vi "DAQAssist-SimulatedSignal.vi"(0 "reference":refnum<vi>, 1 "Stbd Cluster":T2, 2 "Port Cluster":T2, 3 "Corner Cluster Stbd":T1, 4 "Corner Cluster Port":T1) -> (5 "Dynamic Data":dynamicdata(waveform))   [LabVIEW 2012]
uses:
  <vilib>/Analysis/NI_AALPro.lvlib
panel:
  out "x*y":dbl[](array[numeric])
  out "Waveform Graph 2":dynamicdata(graph)
  out "Waveform Graph 3":dynamicdata(graph)
  out "Waveform Graph":dynamicdata(graph)
  out "Frequency Port":dbl
  out "Frequency Stbd":dbl
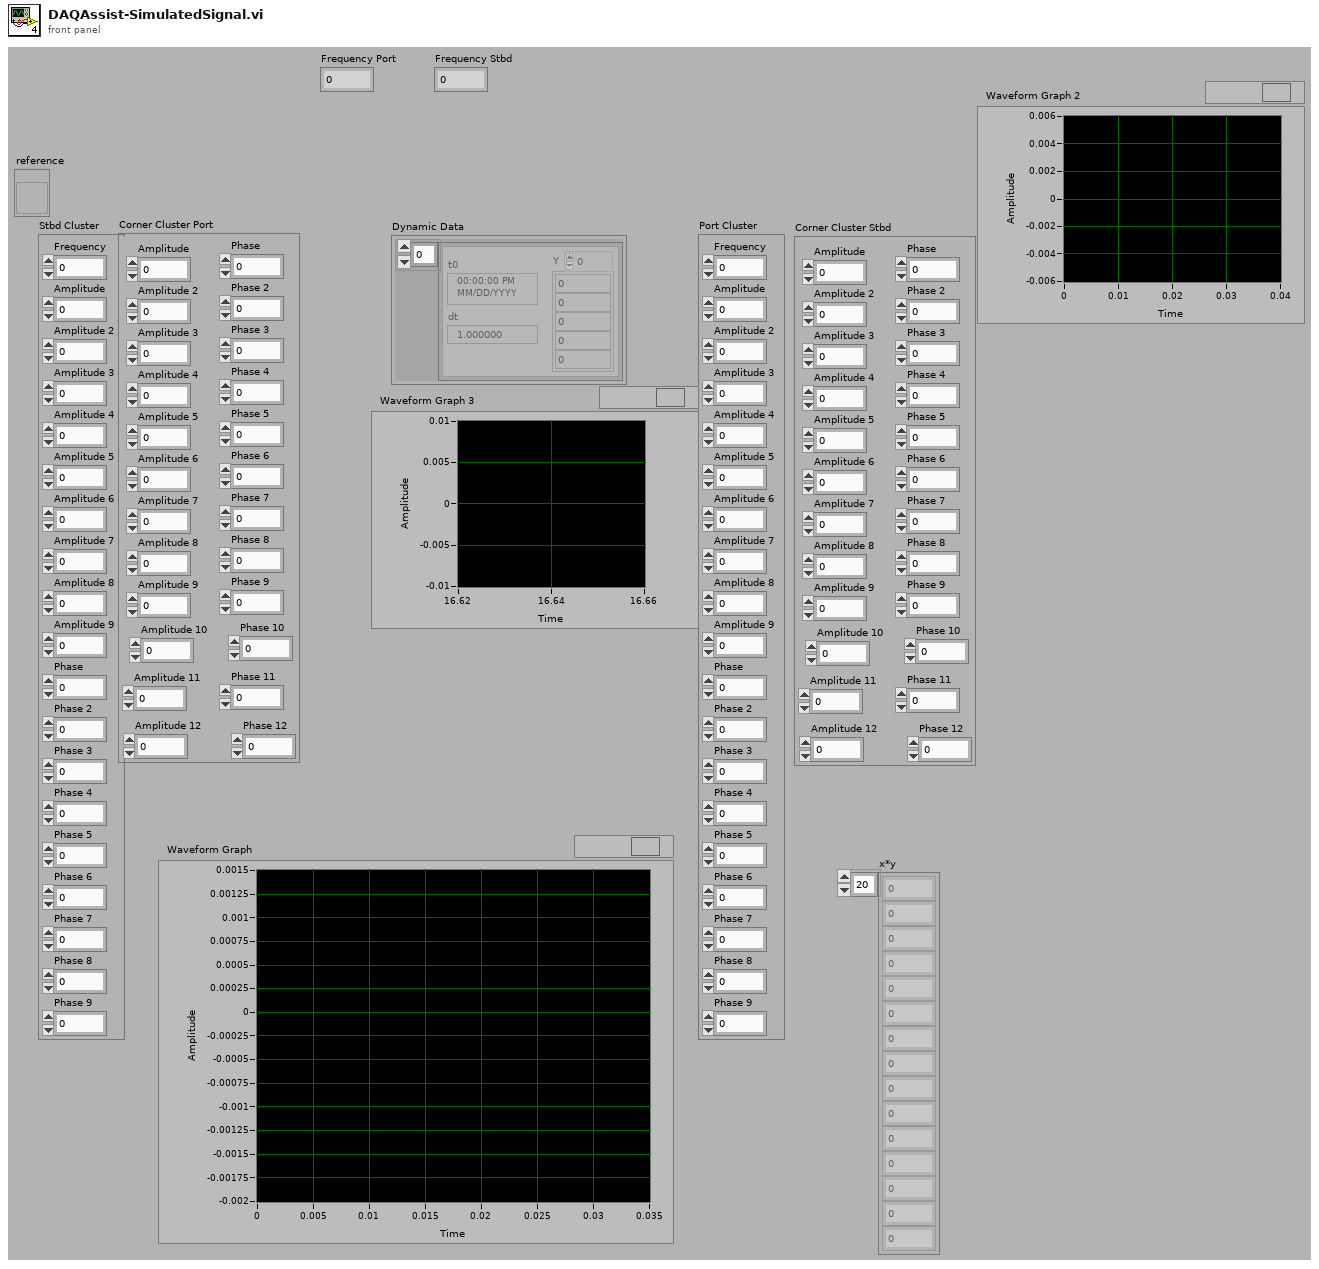
[diagram p1: front panel]
types:
  T1 = cluster{"Amplitude":dbl, "Phase":dbl, "Amplitude 2":dbl, "Phase 2":dbl, "Amplitude 3":dbl, "Phase 3":dbl, "Amplitude 4":dbl, "Phase 4":dbl, "Amplitude 5":dbl, "Phase 5":dbl, "Amplitude 6":dbl, "Phase 6":dbl, "Amplitude 7":dbl, "Phase 7":dbl, "Amplitude 8":dbl, "Phase 8":dbl, "Amplitude 9":dbl, "Phase 9":dbl, "Amplitude 10":dbl, "Phase 10":dbl, "Amplitude 11":dbl, "Phase 11":dbl, "Amplitude 12":dbl, "Phase 12":dbl}
  T2 = cluster{"Frequency":dbl, "Amplitude":dbl, "Amplitude 2":dbl, "Amplitude 3":dbl, "Amplitude 4":dbl, "Amplitude 5":dbl, "Amplitude 6":dbl, "Amplitude 7":dbl, "Amplitude 8":dbl, "Amplitude 9":dbl, "Phase":dbl, "Phase 2":dbl, "Phase 3":dbl, "Phase 4":dbl, "Phase 5":dbl, "Phase 6":dbl, "Phase 7":dbl, "Phase 8":dbl, "Phase 9":dbl}
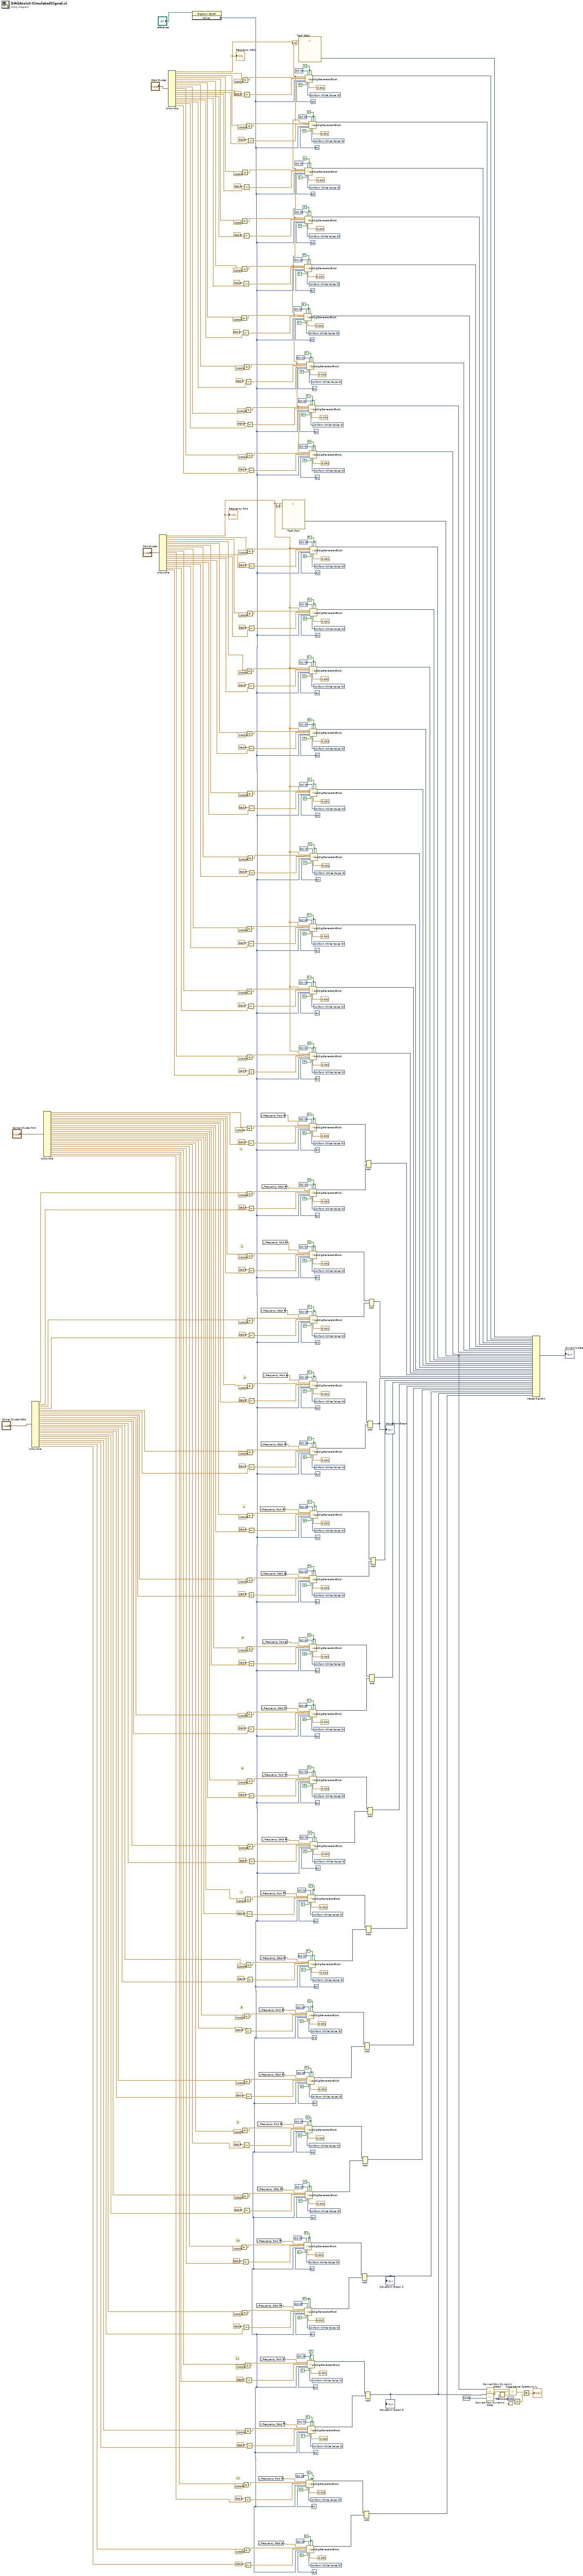
[diagram p0: block diagram]
diagram:
  w12 = TRUE ("Generate Data in Real Time")
  w13 = TRUE ("Generate Data in Real Time")
  w64 = TRUE ("Generate Data in Real Time")
  w65 = TRUE ("Generate Data in Real Time")
  w66 = TRUE ("Generate Data in Real Time")
  w67 = TRUE ("Noise")
  w94 = TRUE ("Generate Data in Real Time")
  w88 = u16 0 items=["DC", "Sine", "Square", "Triangle", "Sawtooth"] ("Generate")
  w89 = u16 0 items=["Uniform White Noise", "Gaussian White Noise", "Periodic Random Noise", "Gamma Noise", "Poisson Noise", "Binomial Noise", "Bernoulli Noise", "MLS Sequence "] ("Noise Ring")
  w100 = u16 0 items=["DC", "Sine", "Square", "Triangle", "Sawtooth"] ("Generate")
  w99 = u16 0 items=["Uniform White Noise", "Gaussian White Noise", "Periodic Random Noise", "Gamma Noise", "Poisson Noise", "Binomial Noise", "Bernoulli Noise", "MLS Sequence "] ("Noise Ring")
  w113 = TRUE ("Generate Data in Real Time")
  w119 = u16 0 items=["DC", "Sine", "Square", "Triangle", "Sawtooth"] ("Generate")
  w118 = u16 0 items=["Uniform White Noise", "Gaussian White Noise", "Periodic Random Noise", "Gamma Noise", "Poisson Noise", "Binomial Noise", "Bernoulli Noise", "MLS Sequence "] ("Noise Ring")
  w107 = u16 0 items=["DC", "Sine", "Square", "Triangle", "Sawtooth"] ("Generate")
  w108 = u16 0 items=["Uniform White Noise", "Gaussian White Noise", "Periodic Random Noise", "Gamma Noise", "Poisson Noise", "Binomial Noise", "Bernoulli Noise", "MLS Sequence "] ("Noise Ring")
  w140 = TRUE ("Generate Data in Real Time")
  w134 = u16 0 items=["DC", "Sine", "Square", "Triangle", "Sawtooth"] ("Generate")
  w135 = u16 0 items=["Uniform White Noise", "Gaussian White Noise", "Periodic Random Noise", "Gamma Noise", "Poisson Noise", "Binomial Noise", "Bernoulli Noise", "MLS Sequence "] ("Noise Ring")
  w146 = u16 0 items=["DC", "Sine", "Square", "Triangle", "Sawtooth"] ("Generate")
  w145 = u16 0 items=["Uniform White Noise", "Gaussian White Noise", "Periodic Random Noise", "Gamma Noise", "Poisson Noise", "Binomial Noise", "Bernoulli Noise", "MLS Sequence "] ("Noise Ring")
  w159 = TRUE ("Generate Data in Real Time")
  w165 = u16 0 items=["DC", "Sine", "Square", "Triangle", "Sawtooth"] ("Generate")
  w164 = u16 0 items=["Uniform White Noise", "Gaussian White Noise", "Periodic Random Noise", "Gamma Noise", "Poisson Noise", "Binomial Noise", "Bernoulli Noise", "MLS Sequence "] ("Noise Ring")
  w153 = u16 0 items=["DC", "Sine", "Square", "Triangle", "Sawtooth"] ("Generate")
  w154 = u16 0 items=["Uniform White Noise", "Gaussian White Noise", "Periodic Random Noise", "Gamma Noise", "Poisson Noise", "Binomial Noise", "Bernoulli Noise", "MLS Sequence "] ("Noise Ring")
  w186 = TRUE ("Generate Data in Real Time")
  w180 = u16 0 items=["DC", "Sine", "Square", "Triangle", "Sawtooth"] ("Generate")
  w181 = u16 0 items=["Uniform White Noise", "Gaussian White Noise", "Periodic Random Noise", "Gamma Noise", "Poisson Noise", "Binomial Noise", "Bernoulli Noise", "MLS Sequence "] ("Noise Ring")
  w192 = u16 0 items=["DC", "Sine", "Square", "Triangle", "Sawtooth"] ("Generate")
  w191 = u16 0 items=["Uniform White Noise", "Gaussian White Noise", "Periodic Random Noise", "Gamma Noise", "Poisson Noise", "Binomial Noise", "Bernoulli Noise", "MLS Sequence "] ("Noise Ring")
  w205 = TRUE ("Generate Data in Real Time")
  w211 = u16 0 items=["DC", "Sine", "Square", "Triangle", "Sawtooth"] ("Generate")
  w210 = u16 0 items=["Uniform White Noise", "Gaussian White Noise", "Periodic Random Noise", "Gamma Noise", "Poisson Noise", "Binomial Noise", "Bernoulli Noise", "MLS Sequence "] ("Noise Ring")
  w199 = u16 0 items=["DC", "Sine", "Square", "Triangle", "Sawtooth"] ("Generate")
  w200 = u16 0 items=["Uniform White Noise", "Gaussian White Noise", "Periodic Random Noise", "Gamma Noise", "Poisson Noise", "Binomial Noise", "Bernoulli Noise", "MLS Sequence "] ("Noise Ring")
  w253 = TRUE ("Generate Data in Real Time")
  w247 = u16 0 items=["DC", "Sine", "Square", "Triangle", "Sawtooth"] ("Generate")
  w248 = u16 0 items=["Uniform White Noise", "Gaussian White Noise", "Periodic Random Noise", "Gamma Noise", "Poisson Noise", "Binomial Noise", "Bernoulli Noise", "MLS Sequence "] ("Noise Ring")
  w254 = TRUE ("Generate Data in Real Time")
  w260 = u16 0 items=["DC", "Sine", "Square", "Triangle", "Sawtooth"] ("Generate")
  w259 = u16 0 items=["Uniform White Noise", "Gaussian White Noise", "Periodic Random Noise", "Gamma Noise", "Poisson Noise", "Binomial Noise", "Bernoulli Noise", "MLS Sequence "] ("Noise Ring")
  w273 = TRUE ("Generate Data in Real Time")
  w267 = u16 0 items=["DC", "Sine", "Square", "Triangle", "Sawtooth"] ("Generate")
  w268 = u16 0 items=["Uniform White Noise", "Gaussian White Noise", "Periodic Random Noise", "Gamma Noise", "Poisson Noise", "Binomial Noise", "Bernoulli Noise", "MLS Sequence "] ("Noise Ring")
  w274 = TRUE ("Generate Data in Real Time")
  w280 = u16 0 items=["DC", "Sine", "Square", "Triangle", "Sawtooth"] ("Generate")
  w279 = u16 0 items=["Uniform White Noise", "Gaussian White Noise", "Periodic Random Noise", "Gamma Noise", "Poisson Noise", "Binomial Noise", "Bernoulli Noise", "MLS Sequence "] ("Noise Ring")
  w293 = TRUE ("Generate Data in Real Time")
  w287 = u16 0 items=["DC", "Sine", "Square", "Triangle", "Sawtooth"] ("Generate")
  w288 = u16 0 items=["Uniform White Noise", "Gaussian White Noise", "Periodic Random Noise", "Gamma Noise", "Poisson Noise", "Binomial Noise", "Bernoulli Noise", "MLS Sequence "] ("Noise Ring")
  w294 = TRUE ("Generate Data in Real Time")
  w300 = u16 0 items=["DC", "Sine", "Square", "Triangle", "Sawtooth"] ("Generate")
  w299 = u16 0 items=["Uniform White Noise", "Gaussian White Noise", "Periodic Random Noise", "Gamma Noise", "Poisson Noise", "Binomial Noise", "Bernoulli Noise", "MLS Sequence "] ("Noise Ring")
  w313 = TRUE ("Generate Data in Real Time")
  w307 = u16 0 items=["DC", "Sine", "Square", "Triangle", "Sawtooth"] ("Generate")
  w308 = u16 0 items=["Uniform White Noise", "Gaussian White Noise", "Periodic Random Noise", "Gamma Noise", "Poisson Noise", "Binomial Noise", "Bernoulli Noise", "MLS Sequence "] ("Noise Ring")
  w314 = TRUE ("Generate Data in Real Time")
  w320 = u16 0 items=["DC", "Sine", "Square", "Triangle", "Sawtooth"] ("Generate")
  w319 = u16 0 items=["Uniform White Noise", "Gaussian White Noise", "Periodic Random Noise", "Gamma Noise", "Poisson Noise", "Binomial Noise", "Bernoulli Noise", "MLS Sequence "] ("Noise Ring")
  w333 = TRUE ("Generate Data in Real Time")
  w327 = u16 0 items=["DC", "Sine", "Square", "Triangle", "Sawtooth"] ("Generate")
  w328 = u16 0 items=["Uniform White Noise", "Gaussian White Noise", "Periodic Random Noise", "Gamma Noise", "Poisson Noise", "Binomial Noise", "Bernoulli Noise", "MLS Sequence "] ("Noise Ring")
  w334 = TRUE ("Generate Data in Real Time")
  w340 = u16 0 items=["DC", "Sine", "Square", "Triangle", "Sawtooth"] ("Generate")
  w339 = u16 0 items=["Uniform White Noise", "Gaussian White Noise", "Periodic Random Noise", "Gamma Noise", "Poisson Noise", "Binomial Noise", "Bernoulli Noise", "MLS Sequence "] ("Noise Ring")
  w353 = TRUE ("Generate Data in Real Time")
  w347 = u16 0 items=["DC", "Sine", "Square", "Triangle", "Sawtooth"] ("Generate")
  w348 = u16 0 items=["Uniform White Noise", "Gaussian White Noise", "Periodic Random Noise", "Gamma Noise", "Poisson Noise", "Binomial Noise", "Bernoulli Noise", "MLS Sequence "] ("Noise Ring")
  w354 = TRUE ("Generate Data in Real Time")
  w360 = u16 0 items=["DC", "Sine", "Square", "Triangle", "Sawtooth"] ("Generate")
  w359 = u16 0 items=["Uniform White Noise", "Gaussian White Noise", "Periodic Random Noise", "Gamma Noise", "Poisson Noise", "Binomial Noise", "Bernoulli Noise", "MLS Sequence "] ("Noise Ring")
  w401 = TRUE ("Generate Data in Real Time")
  w395 = u16 0 items=["DC", "Sine", "Square", "Triangle", "Sawtooth"] ("Generate")
  w396 = u16 0 items=["Uniform White Noise", "Gaussian White Noise", "Periodic Random Noise", "Gamma Noise", "Poisson Noise", "Binomial Noise", "Bernoulli Noise", "MLS Sequence "] ("Noise Ring")
  w402 = TRUE ("Generate Data in Real Time")
  w408 = u16 0 items=["DC", "Sine", "Square", "Triangle", "Sawtooth"] ("Generate")
  w407 = u16 0 items=["Uniform White Noise", "Gaussian White Noise", "Periodic Random Noise", "Gamma Noise", "Poisson Noise", "Binomial Noise", "Bernoulli Noise", "MLS Sequence "] ("Noise Ring")
  w421 = TRUE ("Generate Data in Real Time")
  w415 = u16 0 items=["DC", "Sine", "Square", "Triangle", "Sawtooth"] ("Generate")
  w416 = u16 0 items=["Uniform White Noise", "Gaussian White Noise", "Periodic Random Noise", "Gamma Noise", "Poisson Noise", "Binomial Noise", "Bernoulli Noise", "MLS Sequence "] ("Noise Ring")
  w422 = TRUE ("Generate Data in Real Time")
  w428 = u16 0 items=["DC", "Sine", "Square", "Triangle", "Sawtooth"] ("Generate")
  w427 = u16 0 items=["Uniform White Noise", "Gaussian White Noise", "Periodic Random Noise", "Gamma Noise", "Poisson Noise", "Binomial Noise", "Bernoulli Noise", "MLS Sequence "] ("Noise Ring")
  w441 = TRUE ("Generate Data in Real Time")
  w435 = u16 0 items=["DC", "Sine", "Square", "Triangle", "Sawtooth"] ("Generate")
  w436 = u16 0 items=["Uniform White Noise", "Gaussian White Noise", "Periodic Random Noise", "Gamma Noise", "Poisson Noise", "Binomial Noise", "Bernoulli Noise", "MLS Sequence "] ("Noise Ring")
  w442 = TRUE ("Generate Data in Real Time")
  w448 = u16 0 items=["DC", "Sine", "Square", "Triangle", "Sawtooth"] ("Generate")
  w447 = u16 0 items=["Uniform White Noise", "Gaussian White Noise", "Periodic Random Noise", "Gamma Noise", "Poisson Noise", "Binomial Noise", "Bernoulli Noise", "MLS Sequence "] ("Noise Ring")
  w461 = TRUE ("Generate Data in Real Time")
  w455 = u16 0 items=["DC", "Sine", "Square", "Triangle", "Sawtooth"] ("Generate")
  w456 = u16 0 items=["Uniform White Noise", "Gaussian White Noise", "Periodic Random Noise", "Gamma Noise", "Poisson Noise", "Binomial Noise", "Bernoulli Noise", "MLS Sequence "] ("Noise Ring")
  w462 = TRUE ("Generate Data in Real Time")
  w468 = u16 0 items=["DC", "Sine", "Square", "Triangle", "Sawtooth"] ("Generate")
  w467 = u16 0 items=["Uniform White Noise", "Gaussian White Noise", "Periodic Random Noise", "Gamma Noise", "Poisson Noise", "Binomial Noise", "Bernoulli Noise", "MLS Sequence "] ("Noise Ring")
  w481 = TRUE ("Generate Data in Real Time")
  w475 = u16 0 items=["DC", "Sine", "Square", "Triangle", "Sawtooth"] ("Generate")
  w476 = u16 0 items=["Uniform White Noise", "Gaussian White Noise", "Periodic Random Noise", "Gamma Noise", "Poisson Noise", "Binomial Noise", "Bernoulli Noise", "MLS Sequence "] ("Noise Ring")
  w484 = TRUE ("Generate Data in Real Time")
  w515 = u16 0 items=["DC", "Sine", "Square", "Triangle", "Sawtooth"] ("Generate")
  w514 = u16 0 items=["Uniform White Noise", "Gaussian White Noise", "Periodic Random Noise", "Gamma Noise", "Poisson Noise", "Binomial Noise", "Bernoulli Noise", "MLS Sequence "] ("Noise Ring")
  w527 = TRUE ("Generate Data in Real Time")
  w522 = u16 0 items=["DC", "Sine", "Square", "Triangle", "Sawtooth"] ("Generate")
  w523 = u16 0 items=["Uniform White Noise", "Gaussian White Noise", "Periodic Random Noise", "Gamma Noise", "Poisson Noise", "Binomial Noise", "Bernoulli Noise", "MLS Sequence "] ("Noise Ring")
  w530 = TRUE ("Generate Data in Real Time")
  w535 = u16 0 items=["DC", "Sine", "Square", "Triangle", "Sawtooth"] ("Generate")
  w534 = u16 0 items=["Uniform White Noise", "Gaussian White Noise", "Periodic Random Noise", "Gamma Noise", "Poisson Noise", "Binomial Noise", "Bernoulli Noise", "MLS Sequence "] ("Noise Ring")
  w547 = TRUE ("Generate Data in Real Time")
  w542 = u16 0 items=["DC", "Sine", "Square", "Triangle", "Sawtooth"] ("Generate")
  w543 = u16 0 items=["Uniform White Noise", "Gaussian White Noise", "Periodic Random Noise", "Gamma Noise", "Poisson Noise", "Binomial Noise", "Bernoulli Noise", "MLS Sequence "] ("Noise Ring")
  w550 = TRUE ("Generate Data in Real Time")
  w555 = u16 0 items=["DC", "Sine", "Square", "Triangle", "Sawtooth"] ("Generate")
  w554 = u16 0 items=["Uniform White Noise", "Gaussian White Noise", "Periodic Random Noise", "Gamma Noise", "Poisson Noise", "Binomial Noise", "Bernoulli Noise", "MLS Sequence "] ("Noise Ring")
  w567 = TRUE ("Generate Data in Real Time")
  w562 = u16 0 items=["DC", "Sine", "Square", "Triangle", "Sawtooth"] ("Generate")
  w563 = u16 0 items=["Uniform White Noise", "Gaussian White Noise", "Periodic Random Noise", "Gamma Noise", "Poisson Noise", "Binomial Noise", "Bernoulli Noise", "MLS Sequence "] ("Noise Ring")
  w570 = TRUE ("Generate Data in Real Time")
  w575 = u16 0 items=["DC", "Sine", "Square", "Triangle", "Sawtooth"] ("Generate")
  w574 = u16 0 items=["Uniform White Noise", "Gaussian White Noise", "Periodic Random Noise", "Gamma Noise", "Poisson Noise", "Binomial Noise", "Bernoulli Noise", "MLS Sequence "] ("Noise Ring")
  w587 = TRUE ("Generate Data in Real Time")
  w582 = u16 0 items=["DC", "Sine", "Square", "Triangle", "Sawtooth"] ("Generate")
  w583 = u16 0 items=["Uniform White Noise", "Gaussian White Noise", "Periodic Random Noise", "Gamma Noise", "Poisson Noise", "Binomial Noise", "Bernoulli Noise", "MLS Sequence "] ("Noise Ring")
  w592 = TRUE ("Generate Data in Real Time")
  w597 = u16 0 items=["DC", "Sine", "Square", "Triangle", "Sawtooth"] ("Generate")
  w596 = u16 0 items=["Uniform White Noise", "Gaussian White Noise", "Periodic Random Noise", "Gamma Noise", "Poisson Noise", "Binomial Noise", "Bernoulli Noise", "MLS Sequence "] ("Noise Ring")
  # "12"
  # "11"
  # "10"
  # "9"
  # "8"
  # "7"
  # "6"
  # "5"
  # "4"
  # "3"
  # "2"
  # "1"
  n1 = Unbundle("Corner Cluster Stbd") -> ("Amplitude"=w37:dbl, "Phase"=w36:dbl, "Amplitude 2"=w35:dbl, "Phase 2"=w34:dbl, "Amplitude 3"=w33:dbl, "Phase 3"=w32:dbl, "Amplitude 4"=w31:dbl, "Phase 4"=w30:dbl, "Amplitude 5"=w29:dbl, "Phase 5"=w28:dbl, "Amplitude 6"=w27:dbl, "Phase 6"=w26:dbl, "Amplitude 7"=w25:dbl, "Phase 7"=w24:dbl, "Amplitude 8"=w23:dbl, "Phase 8"=w22:dbl, "Amplitude 9"=w21:dbl, "Phase 9"=w20:dbl, "Amplitude 10"=w19:dbl, "Phase 10"=w18:dbl, "Amplitude 11"=w17:dbl, "Phase 11"=w16:dbl, "Amplitude 12"=w15:dbl, "Phase 12"=w14:dbl)
  n2 = Unbundle("Corner Cluster Port") -> ("Amplitude"=w61:dbl, "Phase"=w60:dbl, "Amplitude 2"=w58:dbl, "Phase 2"=w59:dbl, "Amplitude 3"=w57:dbl, "Phase 3"=w56:dbl, "Amplitude 4"=w55:dbl, "Phase 4"=w54:dbl, "Amplitude 5"=w53:dbl, "Phase 5"=w52:dbl, "Amplitude 6"=w51:dbl, "Phase 6"=w50:dbl, "Amplitude 7"=w49:dbl, "Phase 7"=w48:dbl, "Amplitude 8"=w47:dbl, "Phase 8"=w46:dbl, "Amplitude 9"=w45:dbl, "Phase 9"=w44:dbl, "Amplitude 10"=w43:dbl, "Phase 10"=w42:dbl, "Amplitude 11"=w41:dbl, "Phase 11"=w40:dbl, "Amplitude 12"=w39:dbl, "Phase 12"=w38:dbl)
  n3 = Unbundle("Port Cluster") -> ("Frequency"=w389:dbl, "Amplitude"=w391:dbl, "Amplitude 2"=w379:dbl, "Amplitude 3"=w377:dbl, "Amplitude 4"=w375:dbl, "Amplitude 5"=w373:dbl, "Amplitude 6"=w371:dbl, "Amplitude 7"=w369:dbl, "Amplitude 8"=w367:dbl, "Amplitude 9"=w365:dbl, "Phase"=w390:dbl, "Phase 2"=w378:dbl, "Phase 3"=w376:dbl, "Phase 4"=w374:dbl, "Phase 5"=w372:dbl, "Phase 6"=w370:dbl, "Phase 7"=w368:dbl, "Phase 8"=w366:dbl, "Phase 9"=w364:dbl)
  "Frequency Port" <- w389
  n4 = Unbundle("Stbd Cluster") -> ("Frequency"=w492:dbl, "Amplitude"=w503:dbl, "Amplitude 2"=w502:dbl, "Amplitude 3"=w501:dbl, "Amplitude 4"=w500:dbl, "Amplitude 5"=w499:dbl, "Amplitude 6"=w498:dbl, "Amplitude 7"=w497:dbl, "Amplitude 8"=w496:dbl, "Amplitude 9"=w494:dbl, "Phase"=w589:dbl, "Phase 2"=w509:dbl, "Phase 3"=w508:dbl, "Phase 4"=w507:dbl, "Phase 5"=w506:dbl, "Phase 6"=w505:dbl, "Phase 7"=w504:dbl, "Phase 8"=w495:dbl, "Phase 9"=w493:dbl)
  "Frequency Stbd" <- w492
  n5 = property class="DigNum (strict)"(reference="reference") -> ("Value"=w80:i32)  [unwired: 1 in, 2 out]
  n6 = Divide(x=w498, y=1000.0) -> (x/y=w548:dbl)
  n7 = Divide(x=w43, y=1000.0) -> (x/y=w141:dbl)
  n8 = Divide(x=w499, y=1000.0) -> (x/y=w549:dbl)
  n9 = Divide(x=w19, y=1000.0) -> (x/y=w139:dbl)
  n10 = Divide(x=w500, y=1000.0) -> (x/y=w568:dbl)
  n11 = Divide(x=w45, y=1000.0) -> (x/y=w158:dbl)
  n12 = Divide(x=w501, y=1000.0) -> (x/y=w569:dbl)
  n13 = Divide(x=w503, y=1000.0) -> (x/y=w590:dbl)
  n14 = Divide(x=w21, y=1000.0) -> (x/y=w160:dbl)
  n15 = Subtract(x=360.0, y=w505) -> (x-y=w541:dbl)
  n16 = Subtract(x=360.0, y=w42) -> (x-y=w147:dbl)
  n17 = Divide(x=w39, y=1000.0) -> (x/y=w95:dbl)
  n18 = Subtract(x=360.0, y=w506) -> (x-y=w556:dbl)
  n19 = Subtract(x=360.0, y=w18) -> (x-y=w133:dbl)
  n20 = Subtract(x=360.0, y=w507) -> (x-y=w561:dbl)
  n21 = Divide(x=w47, y=1000.0) -> (x/y=w187:dbl)
  n22 = Subtract(x=360.0, y=w44) -> (x-y=w152:dbl)
  n23 = Divide(x=w15, y=1000.0) -> (x/y=w93:dbl)
  n24 = Subtract(x=360.0, y=w508) -> (x-y=w576:dbl)
  n25 = Divide(x=w497, y=1000.0) -> (x/y=w529:dbl)
  n26 = Subtract(x=360.0, y=w589) -> (x-y=w600:dbl)
  n27 = Divide(x=w23, y=1000.0) -> (x/y=w185:dbl)
  n28 = Subtract(x=360.0, y=w20) -> (x-y=w166:dbl)
  n29 = Divide(x=w41, y=1000.0) -> (x/y=w112:dbl)
  n30 = Subtract(x=360.0, y=w38) -> (x-y=w101:dbl)
  n31 = Divide(x=w49, y=1000.0) -> (x/y=w204:dbl)
  n32 = Divide(x=w17, y=1000.0) -> (x/y=w114:dbl)
  n33 = Subtract(x=360.0, y=w46) -> (x-y=w193:dbl)
  n34 = Subtract(x=360.0, y=w14) -> (x-y=w87:dbl)
  n35 = Subtract(x=360.0, y=w504) -> (x-y=w536:dbl)
  n36 = Divide(x=w496, y=1000.0) -> (x/y=w528:dbl)
  n37 = Divide(x=w25, y=1000.0) -> (x/y=w206:dbl)
  n38 = Subtract(x=360.0, y=w22) -> (x-y=w179:dbl)
  n39 = Divide(x=w502, y=1000.0) -> (x/y=w588:dbl)
  n40 = Subtract(x=360.0, y=w40) -> (x-y=w106:dbl)
  n41 = Divide(x=w377, y=1000.0) -> (x/y=w460:dbl)
  n42 = Divide(x=w369, y=1000.0) -> (x/y=w420:dbl)
  n43 = Divide(x=w367, y=1000.0) -> (x/y=w403:dbl)
  n44 = Divide(x=w61, y=1000.0) -> (x/y=w355:dbl)
  n45 = Divide(x=w29, y=1000.0) -> (x/y=w272:dbl)
  n46 = Divide(x=w494, y=1000.0) -> (x/y=w510:dbl)
  n47 = Divide(x=w375, y=1000.0) -> (x/y=w443:dbl)
  n48 = Divide(x=w365, y=1000.0) -> (x/y=w400:dbl)
  n49 = Divide(x=w37, y=1000.0) -> (x/y=w352:dbl)
  n50 = Divide(x=w58, y=1000.0) -> (x/y=w335:dbl)
  n51 = Divide(x=w31, y=1000.0) -> (x/y=w292:dbl)
  n52 = Divide(x=w53, y=1000.0) -> (x/y=w275:dbl)
  n53 = Divide(x=w51, y=1000.0) -> (x/y=w255:dbl)
  n54 = Subtract(x=360.0, y=w48) -> (x-y=w198:dbl)
  n55 = Subtract(x=360.0, y=w16) -> (x-y=w120:dbl)
  n56 = Divide(x=w391, y=1000.0) -> (x/y=w480:dbl)
  n57 = Divide(x=w379, y=1000.0) -> (x/y=w463:dbl)
  n58 = Divide(x=w373, y=1000.0) -> (x/y=w440:dbl)
  n59 = Divide(x=w35, y=1000.0) -> (x/y=w332:dbl)
  n60 = Divide(x=w57, y=1000.0) -> (x/y=w315:dbl)
  n61 = Divide(x=w33, y=1000.0) -> (x/y=w312:dbl)
  n62 = Divide(x=w55, y=1000.0) -> (x/y=w295:dbl)
  n63 = Subtract(x=360.0, y=w495) -> (x-y=w521:dbl)
  n64 = Divide(x=w371, y=1000.0) -> (x/y=w423:dbl)
  n65 = Divide(x=w27, y=1000.0) -> (x/y=w252:dbl)
  n66 = Subtract(x=360.0, y=w24) -> (x-y=w212:dbl)
  n67 = Subtract(x=360.0, y=w509) -> (x-y=w581:dbl)
  n68 = Subtract(x=360.0, y=w376) -> (x-y=w454:dbl)
  n69 = Subtract(x=360.0, y=w368) -> (x-y=w414:dbl)
  n70 = Subtract(x=360.0, y=w366) -> (x-y=w409:dbl)
  n71 = Subtract(x=360.0, y=w60) -> (x-y=w361:dbl)
  n72 = Subtract(x=360.0, y=w28) -> (x-y=w266:dbl)
  n73 = Subtract(x=360.0, y=w493) -> (x-y=w516:dbl)
  n74 = Subtract(x=360.0, y=w374) -> (x-y=w449:dbl)
  n75 = Subtract(x=360.0, y=w364) -> (x-y=w394:dbl)
  n76 = Subtract(x=360.0, y=w36) -> (x-y=w346:dbl)
  n77 = Subtract(x=360.0, y=w59) -> (x-y=w341:dbl)
  n78 = Subtract(x=360.0, y=w30) -> (x-y=w286:dbl)
  n79 = Subtract(x=360.0, y=w52) -> (x-y=w281:dbl)
  n80 = Subtract(x=360.0, y=w50) -> (x-y=w261:dbl)
  n81 = Subtract(x=360.0, y=w390) -> (x-y=w474:dbl)
  n82 = Subtract(x=360.0, y=w378) -> (x-y=w469:dbl)
  n83 = Subtract(x=360.0, y=w372) -> (x-y=w434:dbl)
  n84 = Subtract(x=360.0, y=w34) -> (x-y=w326:dbl)
  n85 = Subtract(x=360.0, y=w56) -> (x-y=w321:dbl)
  n86 = Subtract(x=360.0, y=w32) -> (x-y=w306:dbl)
  n87 = Subtract(x=360.0, y=w54) -> (x-y=w301:dbl)
  n88 = Subtract(x=360.0, y=w370) -> (x-y=w429:dbl)
  n89 = Subtract(x=360.0, y=w26) -> (x-y=w246:dbl)
  n90 = local read "Frequency Stbd"() -> (w129:dbl)
  n91 = local read "Frequency Port"() -> (w130:dbl)
  n92 = local read "Frequency Stbd"() -> (w170:dbl)
  n93 = local read "Frequency Port"() -> (w169:dbl)
  n94 = local read "Frequency Stbd"() -> (w83:dbl)
  n95 = local read "Frequency Port"() -> (w84:dbl)
  n96 = local read "Frequency Stbd"() -> (w175:dbl)
  n97 = local read "Frequency Port"() -> (w176:dbl)
  n98 = local read "Frequency Stbd"() -> (w124:dbl)
  n99 = local read "Frequency Port"() -> (w235:dbl)
  n100 = local read "Frequency Port"() -> (w123:dbl)
  n101 = local read "Frequency Stbd"() -> (w216:dbl)
  n102 = local read "Frequency Port"() -> (w215:dbl)
  n103 = local read "Frequency Port"() -> (w243:dbl)
  n104 = local read "Frequency Stbd"() -> (w239:dbl)
  n105 = local read "Frequency Stbd"() -> (w236:dbl)
  n106 = local read "Frequency Stbd"() -> (w234:dbl)
  n107 = local read "Frequency Stbd"() -> (w223:dbl)
  n108 = local read "Frequency Stbd"() -> (w240:dbl)
  n109 = local read "Frequency Stbd"() -> (w222:dbl)
  n110 = local read "Frequency Port"() -> (w224:dbl)
  n111 = local read "Frequency Port"() -> (w238:dbl)
  n112 = local read "Frequency Port"() -> (w225:dbl)
  n113 = local read "Frequency Port"() -> (w237:dbl)
  n114 = call "Tach Port"("Frequency"=w389, "Amplitude"=4.0) -> ("Square"=w10:dynamicdata)  [unwired: 12 in, 1 out]
  n115 = call "Tach Stbd"("Frequency"=w492, "Amplitude"=4.0) -> ("Square"=w598:dynamicdata)  [unwired: 12 in, 1 out]
  n116 = call <vilib>:"subSigGeneratorBlock.vi"("Frequency"=w492, "Amplitude"=w548, "Phase"=w541, "Sampling Rate (Hz)"=w80, "# of Samples"=64, "Noise"=TRUE, "Generate"=w542, "Noise Ring"=w543, "Noise Amplitude"=0.001, "Generate Data in Real Time"=w547, "relative time?"=w547) -> ("Signal"=w487:dynamicdata)  [unwired: 15 in, 1 out]
  n117 = call <vilib>:"subSigGeneratorBlock.vi"("Frequency"=w130, "Amplitude"=w141, "Phase"=w147, "Sampling Rate (Hz)"=w80, "# of Samples"=64, "Noise"=TRUE, "Generate"=w146, "Noise Ring"=w145, "Noise Amplitude"=0.001, "Generate Data in Real Time"=w64, "relative time?"=w64) -> ("Signal"=w128:dynamicdata)  [unwired: 15 in, 1 out]
  n118 = call <vilib>:"subSigGeneratorBlock.vi"("Frequency"=w492, "Amplitude"=w549, "Phase"=w556, "Sampling Rate (Hz)"=w80, "# of Samples"=64, "Noise"=TRUE, "Generate"=w555, "Noise Ring"=w554, "Noise Amplitude"=0.001, "Generate Data in Real Time"=w550, "relative time?"=w550) -> ("Signal"=w488:dynamicdata)  [unwired: 15 in, 1 out]
  n119 = call <vilib>:"subSigGeneratorBlock.vi"("Frequency"=w129, "Amplitude"=w139, "Phase"=w133, "Sampling Rate (Hz)"=w80, "# of Samples"=64, "Noise"=TRUE, "Generate"=w134, "Noise Ring"=w135, "Noise Amplitude"=0.001, "Generate Data in Real Time"=w140, "relative time?"=w140) -> ("Signal"=w127:dynamicdata)  [unwired: 15 in, 1 out]
  n120 = call <vilib>:"subSigGeneratorBlock.vi"("Frequency"=w492, "Amplitude"=w568, "Phase"=w561, "Sampling Rate (Hz)"=w80, "# of Samples"=64, "Noise"=TRUE, "Generate"=w562, "Noise Ring"=w563, "Noise Amplitude"=0.001, "Generate Data in Real Time"=w567, "relative time?"=w567) -> ("Signal"=w489:dynamicdata)  [unwired: 15 in, 1 out]
  n121 = call <vilib>:"subSigGeneratorBlock.vi"("Frequency"=w169, "Amplitude"=w158, "Phase"=w152, "Sampling Rate (Hz)"=w80, "# of Samples"=64, "Noise"=TRUE, "Generate"=w153, "Noise Ring"=w154, "Noise Amplitude"=0.001, "Generate Data in Real Time"=w65, "relative time?"=w65) -> ("Signal"=w171:dynamicdata)  [unwired: 15 in, 1 out]
  n122 = call <vilib>:"subSigGeneratorBlock.vi"("Frequency"=w492, "Amplitude"=w569, "Phase"=w576, "Sampling Rate (Hz)"=w80, "# of Samples"=64, "Noise"=TRUE, "Generate"=w575, "Noise Ring"=w574, "Noise Amplitude"=0.001, "Generate Data in Real Time"=w570, "relative time?"=w570) -> ("Signal"=w490:dynamicdata)  [unwired: 15 in, 1 out]
  n123 = call <vilib>:"subSigGeneratorBlock.vi"("Frequency"=w492, "Amplitude"=w590, "Phase"=w600, "Sampling Rate (Hz)"=w80, "# of Samples"=64, "Noise"=TRUE, "Generate"=w597, "Noise Ring"=w596, "Noise Amplitude"=0.001, "Generate Data in Real Time"=w592, "relative time?"=w592) -> ("Signal"=w591:dynamicdata)  [unwired: 15 in, 1 out]
  n124 = call <vilib>:"subSigGeneratorBlock.vi"("Frequency"=w170, "Amplitude"=w160, "Phase"=w166, "Sampling Rate (Hz)"=w80, "# of Samples"=64, "Noise"=TRUE, "Generate"=w165, "Noise Ring"=w164, "Noise Amplitude"=0.001, "Generate Data in Real Time"=w159, "relative time?"=w159) -> ("Signal"=w172:dynamicdata)  [unwired: 15 in, 1 out]
  n125 = call <vilib>:"subSigGeneratorBlock.vi"("Frequency"=w84, "Amplitude"=w95, "Phase"=w101, "Sampling Rate (Hz)"=w80, "# of Samples"=64, "Noise"=TRUE, "Generate"=w100, "Noise Ring"=w99, "Noise Amplitude"=0.001, "Generate Data in Real Time"=w12, "relative time?"=w12) -> ("Signal"=w82:dynamicdata)  [unwired: 15 in, 1 out]
  n126 = call <vilib>:"subSigGeneratorBlock.vi"("Frequency"=w176, "Amplitude"=w187, "Phase"=w193, "Sampling Rate (Hz)"=w80, "# of Samples"=64, "Noise"=TRUE, "Generate"=w192, "Noise Ring"=w191, "Noise Amplitude"=0.001, "Generate Data in Real Time"=w67, "relative time?"=w67) -> ("Signal"=w174:dynamicdata)  [unwired: 15 in, 1 out]
  n127 = call <vilib>:"subSigGeneratorBlock.vi"("Frequency"=w83, "Amplitude"=w93, "Phase"=w87, "Sampling Rate (Hz)"=w80, "# of Samples"=64, "Noise"=TRUE, "Generate"=w88, "Noise Ring"=w89, "Noise Amplitude"=0.001, "Generate Data in Real Time"=w94, "relative time?"=w94) -> ("Signal"=w81:dynamicdata)  [unwired: 15 in, 1 out]
  n128 = call <vilib>:"subSigGeneratorBlock.vi"("Frequency"=w492, "Amplitude"=w529, "Phase"=w536, "Sampling Rate (Hz)"=w80, "# of Samples"=64, "Noise"=TRUE, "Generate"=w535, "Noise Ring"=w534, "Noise Amplitude"=0.001, "Generate Data in Real Time"=w530, "relative time?"=w530) -> ("Signal"=w486:dynamicdata)  [unwired: 15 in, 1 out]
  n129 = call <vilib>:"subSigGeneratorBlock.vi"("Frequency"=w175, "Amplitude"=w185, "Phase"=w179, "Sampling Rate (Hz)"=w80, "# of Samples"=64, "Noise"=TRUE, "Generate"=w180, "Noise Ring"=w181, "Noise Amplitude"=0.001, "Generate Data in Real Time"=w186, "relative time?"=w186) -> ("Signal"=w173:dynamicdata)  [unwired: 15 in, 1 out]
  n130 = call <vilib>:"subSigGeneratorBlock.vi"("Frequency"=w123, "Amplitude"=w112, "Phase"=w106, "Sampling Rate (Hz)"=w80, "# of Samples"=64, "Noise"=TRUE, "Generate"=w107, "Noise Ring"=w108, "Noise Amplitude"=0.001, "Generate Data in Real Time"=w13, "relative time?"=w13) -> ("Signal"=w125:dynamicdata)  [unwired: 15 in, 1 out]
  n131 = call <vilib>:"subSigGeneratorBlock.vi"("Frequency"=w215, "Amplitude"=w204, "Phase"=w198, "Sampling Rate (Hz)"=w80, "# of Samples"=64, "Noise"=TRUE, "Generate"=w199, "Noise Ring"=w200, "Noise Amplitude"=0.001, "Generate Data in Real Time"=w66, "relative time?"=w66) -> ("Signal"=w217:dynamicdata)  [unwired: 15 in, 1 out]
  n132 = call <vilib>:"subSigGeneratorBlock.vi"("Frequency"=w124, "Amplitude"=w114, "Phase"=w120, "Sampling Rate (Hz)"=w80, "# of Samples"=64, "Noise"=TRUE, "Generate"=w119, "Noise Ring"=w118, "Noise Amplitude"=0.001, "Generate Data in Real Time"=w113, "relative time?"=w113) -> ("Signal"=w126:dynamicdata)  [unwired: 15 in, 1 out]
  n133 = call <vilib>:"subSigGeneratorBlock.vi"("Frequency"=w492, "Amplitude"=w528, "Phase"=w521, "Sampling Rate (Hz)"=w80, "# of Samples"=64, "Noise"=TRUE, "Generate"=w522, "Noise Ring"=w523, "Noise Amplitude"=0.001, "Generate Data in Real Time"=w527, "relative time?"=w527) -> ("Signal"=w485:dynamicdata)  [unwired: 15 in, 1 out]
  n134 = call <vilib>:"subSigGeneratorBlock.vi"("Frequency"=w216, "Amplitude"=w206, "Phase"=w212, "Sampling Rate (Hz)"=w80, "# of Samples"=64, "Noise"=TRUE, "Generate"=w211, "Noise Ring"=w210, "Noise Amplitude"=0.001, "Generate Data in Real Time"=w205, "relative time?"=w205) -> ("Signal"=w218:dynamicdata)  [unwired: 15 in, 1 out]
  n135 = call <vilib>:"subSigGeneratorBlock.vi"("Frequency"=w492, "Amplitude"=w588, "Phase"=w581, "Sampling Rate (Hz)"=w80, "# of Samples"=64, "Noise"=TRUE, "Generate"=w582, "Noise Ring"=w583, "Noise Amplitude"=0.001, "Generate Data in Real Time"=w587, "relative time?"=w587) -> ("Signal"=w491:dynamicdata)  [unwired: 15 in, 1 out]
  n136 = call <vilib>:"subSigGeneratorBlock.vi"("Frequency"=w389, "Amplitude"=w460, "Phase"=w454, "Sampling Rate (Hz)"=w80, "# of Samples"=64, "Noise"=TRUE, "Generate"=w455, "Noise Ring"=w456, "Noise Amplitude"=0.001, "Generate Data in Real Time"=w461, "relative time?"=w461) -> ("Signal"=w382:dynamicdata)  [unwired: 15 in, 1 out]
  n137 = call <vilib>:"subSigGeneratorBlock.vi"("Frequency"=w389, "Amplitude"=w420, "Phase"=w414, "Sampling Rate (Hz)"=w80, "# of Samples"=64, "Noise"=TRUE, "Generate"=w415, "Noise Ring"=w416, "Noise Amplitude"=0.001, "Generate Data in Real Time"=w421, "relative time?"=w421) -> ("Signal"=w386:dynamicdata)  [unwired: 15 in, 1 out]
  n138 = call <vilib>:"subSigGeneratorBlock.vi"("Frequency"=w389, "Amplitude"=w403, "Phase"=w409, "Sampling Rate (Hz)"=w80, "# of Samples"=64, "Noise"=TRUE, "Generate"=w408, "Noise Ring"=w407, "Noise Amplitude"=0.001, "Generate Data in Real Time"=w402, "relative time?"=w402) -> ("Signal"=w387:dynamicdata)  [unwired: 15 in, 1 out]
  n139 = call <vilib>:"subSigGeneratorBlock.vi"("Frequency"=w243, "Amplitude"=w355, "Phase"=w361, "Sampling Rate (Hz)"=w80, "# of Samples"=64, "Noise"=TRUE, "Generate"=w360, "Noise Ring"=w359, "Noise Amplitude"=0.001, "Generate Data in Real Time"=w354, "relative time?"=w354) -> ("Signal"=w242:dynamicdata)  [unwired: 15 in, 1 out]
  n140 = call <vilib>:"subSigGeneratorBlock.vi"("Frequency"=w223, "Amplitude"=w272, "Phase"=w266, "Sampling Rate (Hz)"=w80, "# of Samples"=64, "Noise"=TRUE, "Generate"=w267, "Noise Ring"=w268, "Noise Amplitude"=0.001, "Generate Data in Real Time"=w273, "relative time?"=w273) -> ("Signal"=w226:dynamicdata)  [unwired: 15 in, 1 out]
  n141 = call <vilib>:"subSigGeneratorBlock.vi"("Frequency"=w492, "Amplitude"=w510, "Phase"=w516, "Sampling Rate (Hz)"=w80, "# of Samples"=64, "Noise"=TRUE, "Generate"=w515, "Noise Ring"=w514, "Noise Amplitude"=0.001, "Generate Data in Real Time"=w484, "relative time?"=w484) -> ("Signal"=w483:dynamicdata)  [unwired: 15 in, 1 out]
  n142 = call <vilib>:"subSigGeneratorBlock.vi"("Frequency"=w389, "Amplitude"=w443, "Phase"=w449, "Sampling Rate (Hz)"=w80, "# of Samples"=64, "Noise"=TRUE, "Generate"=w448, "Noise Ring"=w447, "Noise Amplitude"=0.001, "Generate Data in Real Time"=w442, "relative time?"=w442) -> ("Signal"=w383:dynamicdata)  [unwired: 15 in, 1 out]
  n143 = call <vilib>:"subSigGeneratorBlock.vi"("Frequency"=w389, "Amplitude"=w400, "Phase"=w394, "Sampling Rate (Hz)"=w80, "# of Samples"=64, "Noise"=TRUE, "Generate"=w395, "Noise Ring"=w396, "Noise Amplitude"=0.001, "Generate Data in Real Time"=w401, "relative time?"=w401) -> ("Signal"=w388:dynamicdata)  [unwired: 15 in, 1 out]
  n144 = call <vilib>:"subSigGeneratorBlock.vi"("Frequency"=w240, "Amplitude"=w352, "Phase"=w346, "Sampling Rate (Hz)"=w80, "# of Samples"=64, "Noise"=TRUE, "Generate"=w347, "Noise Ring"=w348, "Noise Amplitude"=0.001, "Generate Data in Real Time"=w353, "relative time?"=w353) -> ("Signal"=w241:dynamicdata)  [unwired: 15 in, 1 out]
  n145 = call <vilib>:"subSigGeneratorBlock.vi"("Frequency"=w238, "Amplitude"=w335, "Phase"=w341, "Sampling Rate (Hz)"=w80, "# of Samples"=64, "Noise"=TRUE, "Generate"=w340, "Noise Ring"=w339, "Noise Amplitude"=0.001, "Generate Data in Real Time"=w334, "relative time?"=w334) -> ("Signal"=w233:dynamicdata)  [unwired: 15 in, 1 out]
  n146 = call <vilib>:"subSigGeneratorBlock.vi"("Frequency"=w234, "Amplitude"=w292, "Phase"=w286, "Sampling Rate (Hz)"=w80, "# of Samples"=64, "Noise"=TRUE, "Generate"=w287, "Noise Ring"=w288, "Noise Amplitude"=0.001, "Generate Data in Real Time"=w293, "relative time?"=w293) -> ("Signal"=w228:dynamicdata)  [unwired: 15 in, 1 out]
  n147 = call <vilib>:"subSigGeneratorBlock.vi"("Frequency"=w225, "Amplitude"=w275, "Phase"=w281, "Sampling Rate (Hz)"=w80, "# of Samples"=64, "Noise"=TRUE, "Generate"=w280, "Noise Ring"=w279, "Noise Amplitude"=0.001, "Generate Data in Real Time"=w274, "relative time?"=w274) -> ("Signal"=w227:dynamicdata)  [unwired: 15 in, 1 out]
  n148 = call <vilib>:"subSigGeneratorBlock.vi"("Frequency"=w224, "Amplitude"=w255, "Phase"=w261, "Sampling Rate (Hz)"=w80, "# of Samples"=64, "Noise"=TRUE, "Generate"=w260, "Noise Ring"=w259, "Noise Amplitude"=0.001, "Generate Data in Real Time"=w254, "relative time?"=w254) -> ("Signal"=w221:dynamicdata)  [unwired: 15 in, 1 out]
  n149 = call <vilib>:"subSigGeneratorBlock.vi"("Frequency"=w389, "Amplitude"=w480, "Phase"=w474, "Sampling Rate (Hz)"=w80, "# of Samples"=64, "Noise"=TRUE, "Generate"=w475, "Noise Ring"=w476, "Noise Amplitude"=0.001, "Generate Data in Real Time"=w481, "relative time?"=w481) -> ("Signal"=w380:dynamicdata)  [unwired: 15 in, 1 out]
  n150 = call <vilib>:"subSigGeneratorBlock.vi"("Frequency"=w389, "Amplitude"=w463, "Phase"=w469, "Sampling Rate (Hz)"=w80, "# of Samples"=64, "Noise"=TRUE, "Generate"=w468, "Noise Ring"=w467, "Noise Amplitude"=0.001, "Generate Data in Real Time"=w462, "relative time?"=w462) -> ("Signal"=w381:dynamicdata)  [unwired: 15 in, 1 out]
  n151 = call <vilib>:"subSigGeneratorBlock.vi"("Frequency"=w389, "Amplitude"=w440, "Phase"=w434, "Sampling Rate (Hz)"=w80, "# of Samples"=64, "Noise"=TRUE, "Generate"=w435, "Noise Ring"=w436, "Noise Amplitude"=0.001, "Generate Data in Real Time"=w441, "relative time?"=w441) -> ("Signal"=w384:dynamicdata)  [unwired: 15 in, 1 out]
  n152 = call <vilib>:"subSigGeneratorBlock.vi"("Frequency"=w239, "Amplitude"=w332, "Phase"=w326, "Sampling Rate (Hz)"=w80, "# of Samples"=64, "Noise"=TRUE, "Generate"=w327, "Noise Ring"=w328, "Noise Amplitude"=0.001, "Generate Data in Real Time"=w333, "relative time?"=w333) -> ("Signal"=w232:dynamicdata)  [unwired: 15 in, 1 out]
  n153 = call <vilib>:"subSigGeneratorBlock.vi"("Frequency"=w237, "Amplitude"=w315, "Phase"=w321, "Sampling Rate (Hz)"=w80, "# of Samples"=64, "Noise"=TRUE, "Generate"=w320, "Noise Ring"=w319, "Noise Amplitude"=0.001, "Generate Data in Real Time"=w314, "relative time?"=w314) -> ("Signal"=w231:dynamicdata)  [unwired: 15 in, 1 out]
  n154 = call <vilib>:"subSigGeneratorBlock.vi"("Frequency"=w236, "Amplitude"=w312, "Phase"=w306, "Sampling Rate (Hz)"=w80, "# of Samples"=64, "Noise"=TRUE, "Generate"=w307, "Noise Ring"=w308, "Noise Amplitude"=0.001, "Generate Data in Real Time"=w313, "relative time?"=w313) -> ("Signal"=w230:dynamicdata)  [unwired: 15 in, 1 out]
  n155 = call <vilib>:"subSigGeneratorBlock.vi"("Frequency"=w389, "Amplitude"=w423, "Phase"=w429, "Sampling Rate (Hz)"=w80, "# of Samples"=64, "Noise"=TRUE, "Generate"=w428, "Noise Ring"=w427, "Noise Amplitude"=0.001, "Generate Data in Real Time"=w422, "relative time?"=w422) -> ("Signal"=w385:dynamicdata)  [unwired: 15 in, 1 out]
  n156 = call <vilib>:"subSigGeneratorBlock.vi"("Frequency"=w235, "Amplitude"=w295, "Phase"=w301, "Sampling Rate (Hz)"=w80, "# of Samples"=64, "Noise"=TRUE, "Generate"=w300, "Noise Ring"=w299, "Noise Amplitude"=0.001, "Generate Data in Real Time"=w294, "relative time?"=w294) -> ("Signal"=w229:dynamicdata)  [unwired: 15 in, 1 out]
  n157 = call <vilib>:"subSigGeneratorBlock.vi"("Frequency"=w222, "Amplitude"=w252, "Phase"=w246, "Sampling Rate (Hz)"=w80, "# of Samples"=64, "Noise"=TRUE, "Generate"=w247, "Noise Ring"=w248, "Noise Amplitude"=0.001, "Generate Data in Real Time"=w253, "relative time?"=w253) -> ("Signal"=w220:dynamicdata)  [unwired: 15 in, 1 out]
  n158 = Add(1:w127, 2:w128) -> (0:w69:dynamicdata)  [unwired: 1 in, 1 out]
  "Waveform Graph 2" <- w69
  n159 = Add(1:w172, 2:w171) -> (0:w70:dynamicdata)  [unwired: 1 in, 1 out]
  n160 = Add(1:w81, 2:w82) -> (0:w68:dynamicdata)  [unwired: 1 in, 1 out]
  n161 = Add(1:w173, 2:w174) -> (0:w71:dynamicdata)  [unwired: 1 in, 1 out]
  n162 = Add(1:w126, 2:w125) -> (0:w11:dynamicdata)  [unwired: 1 in, 1 out]
  "Waveform Graph 3" <- w11
  n163 = Add(1:w218, 2:w217) -> (0:w72:dynamicdata)  [unwired: 1 in, 1 out]
  n164 = Add(1:w241, 2:w242) -> (0:w78:dynamicdata)  [unwired: 1 in, 1 out]
  n165 = Add(1:w230, 2:w231) -> (0:w76:dynamicdata)  [unwired: 1 in, 1 out]
  "Waveform Graph" <- w76
  n166 = Add(1:w220, 2:w221) -> (0:w73:dynamicdata)  [unwired: 1 in, 1 out]
  n167 = Add(1:w232, 2:w233) -> (0:w77:dynamicdata)  [unwired: 1 in, 1 out]
  n168 = Add(1:w226, 2:w227) -> (0:w74:dynamicdata)  [unwired: 1 in, 1 out]
  n169 = Add(1:w228, 2:w229) -> (0:w75:dynamicdata)  [unwired: 1 in, 1 out]
  n170 = call "Convert from Dynamic Data"("Dynamic Data Type"=w11) -> ("Array"=w3:dbl[])  [unwired: 3 in]
  n171 = call "Convert from Dynamic Data2"("Dynamic Data Type"=w10) -> ("Array"=w2:dbl[])  [unwired: 3 in]
  n172 = Reciprocal(x=2048 ("Sample Frequency (Hz)")) -> (1/x=w8:dbl)
  n173 = call <vilib>:"Cross Power Spectrum.vi"("dt"=w8, "Signal Y (V)"=w3, "Signal X (V)"=w2) -> ("Cross Power XY Spectrum Phase (radians)"=w7:dbl[])  [unwired: 2 out]
  n174 = Divide(x=180, y=3.141592653589793) -> (x/y=w4:dbl)
  n175 = Multiply(x=w7, y=w4) -> (x*y=→"x*y":dbl[])
  n176 = Merge Signals(w598, w591, w491, w490, w489, w488, w487, w486, w485, w483, w10, w380, w381, w382, w383, w384, w385, w386, w387, w388, w78, w77, w76, w75, w74, w73, w72, w71, w70, w69, w11, w68) -> (→"Dynamic Data":dynamicdata)
